vi "RVC300_open_control.vi"(11 "Enter Flow Rate (mbar*Liters/sec)":dbl) -> (2 "Unacceptable Flow Rate Value":bool, 3 "Valve Percentage Open":dbl)   [LabVIEW 2014]
uses:
  <vilib>/Utility/file.llb/Read From Spreadsheet File (DBL).vi
  <vilib>/DAQmx/create/channels.llb/DAQmx Create Channel (AO-Voltage-Basic).vi
  <vilib>/DAQmx/write.llb/DAQmx Write (Analog DBL 1Chan 1Samp).vi
  <vilib>/gmath/NI_Gmath.lvlib
panel:
  in  "timeout":dbl=10.0 format="%0.2f"
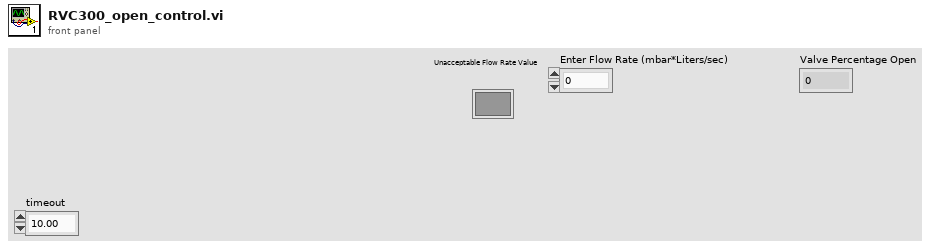
[diagram p1: front panel]
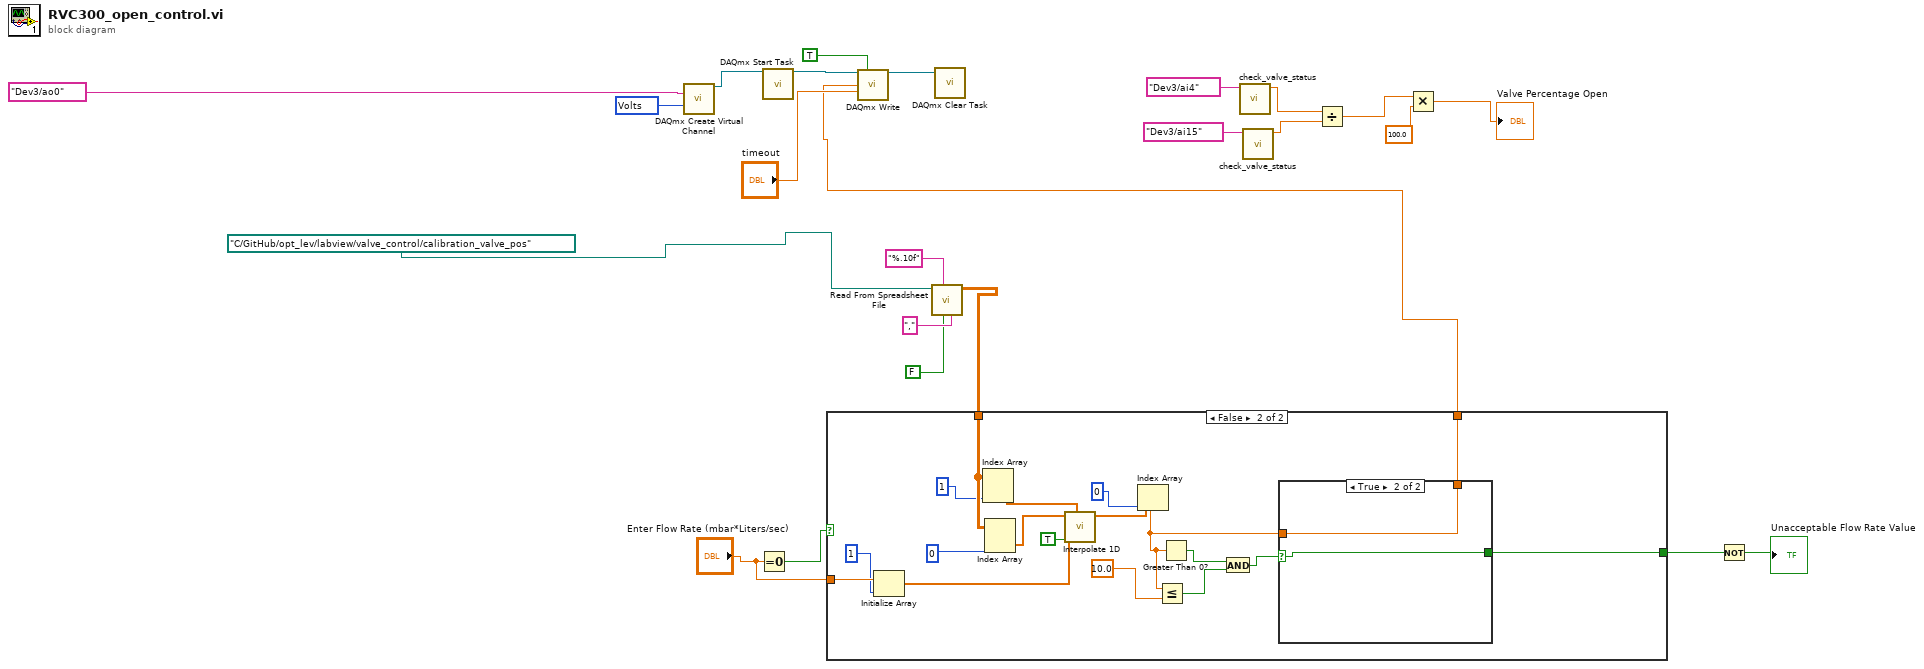
[diagram p0: block diagram]
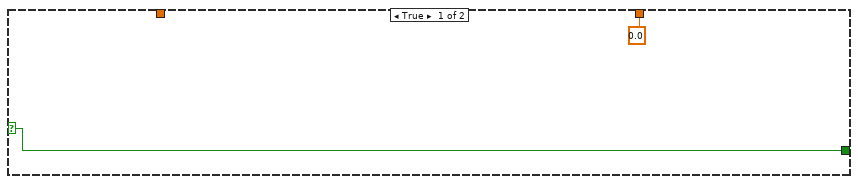
[diagram p2: hidden frame]
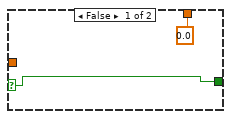
[diagram p3: hidden frame]
diagram:
  w1 = 10348 items=["Volts"=10348, "From Custom Scale"=10065] ("units")
  n1 = call-poly <vilib>:"DAQmx Create Virtual Channel.vi"("physical channels"=tag "Dev3/ao0", "units"=w1) -> ("task out"=w10:refnum<k21>)  [unwired: 12 in, 1 out]
  n2 = Equal To 0?(x="Enter Flow Rate (mbar*Liters/sec)") -> (x = 0?=w3:bool)
  n3 = call <vilib>:"DAQmx Start Task.vi"("task/channels in"=w10) -> ("task out"=w22:refnum<k21>)  [unwired: 13 in, 1 out]
  n4 = call-poly <vilib>:"Read From Spreadsheet File.vi"("delimiter (\\t)"="," ("delimiter (\\t)"), "transpose (no:F)"=FALSE, "format (%.3f)"="%.10f", "file path (dialog if empty)"=path "C:/GitHub/opt_lev/labview/valve_control/calibration_valve_pos" ("input file")) -> ("all rows"=w15:dbl[][])  [unwired: 3 in, 4 out]
  n5 = case shown="False" w3 {
    selector: w3 -> [w25 _]
    tunnel: w15 -> [_ w43]
    tunnel: "Enter Flow Rate (mbar*Liters/sec)" -> [_ w38]
    tunnel: [0.0 ("Numeric") w29] -> w5
    tunnel: [w25 w27] -> w4
    frame True {
    }
    frame False {
      n6 = Initialize Array(w38, 1 ("dimension size")) -> (w36:dbl[])
      n7 = Index Array(array=w43, index (col)=1 ("index (row)")) -> (element=w44:dbl[])  [unwired: 1 in]
      n8 = Index Array(array=w43, index (col)=0 ("index (row)")) -> (element=w42:dbl[])  [unwired: 1 in]
      n9 = call <vilib>:"Interpolate 1D.vi"("X is monotonic"=TRUE, "xi"=w36, "X"=w44, "Y"=w42) -> ("yi"=w32:dbl[])  [unwired: 5 in, 2 out]
      n10 = Index Array(array=w32, index=0) -> (element=w28:dbl)
      n11 = Less Or Equal?(x=w28, y=10.0) -> (x <= y?=w33:bool)
      n12 = Greater Than 0?(x=w28) -> (x > 0?=w34:bool)
      n13 = And(x=w34, y=w33) -> (x .and. y?=w30:bool)
      n14 = case shown="True" w30 {
        selector: w30 -> [w45 w47]
        tunnel: w28 -> [_ w48]
        tunnel: [0.0 ("Numeric") w48] -> w29
        tunnel: [w45 w47] -> w27
        frame False {
        }
        frame True {
        }
      }
    }
  }
  n15 = call-poly <vilib>:"DAQmx Write.vi"("task/channels in"=w22, "auto start"=TRUE, "data"=w5, "timeout"="timeout") -> ("task out"=w19:refnum<k21>)  [unwired: 9 in, 2 out]
  n16 = call <vilib>:"DAQmx Clear Task.vi"("task in"=w19) -> ()  [unwired: 14 in, 1 out]
  n17 = call "check_valve_status.vi"("Channel 1"=tag "Dev3/ai4") -> ("Ch. 1 value"=w12:dbl)  [unwired: 9 in, 1 out]
  n18 = call "check_valve_status.vi"("Channel 1"=tag "Dev3/ai15") -> ("Ch. 1 value"=w11:dbl)  [unwired: 9 in, 1 out]
  n19 = Divide(x=w12, y=w11) -> (x/y=w9:dbl)
  n20 = Multiply(x=w9, y=100.0) -> (x*y=→"Valve Percentage Open":dbl)
  n21 = Not(x=w4) -> (.not. x?=→"Unacceptable Flow Rate Value":bool)
